vi "GetIdxString.vi"(10 "IdxArray":i32[](array[numeric]), 11 "StrArray":string[](array[string])) -> (7 "TrueArray":string[](array[string]))   [LabVIEW 2015]
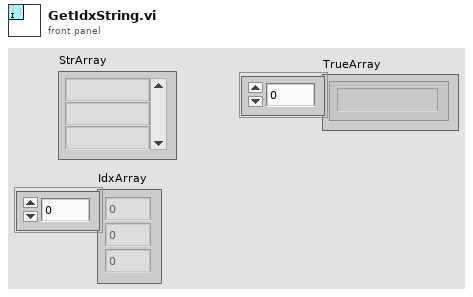
[diagram p1: front panel]
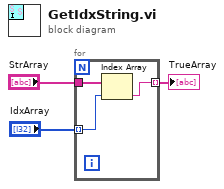
[diagram p0: block diagram]
diagram:
  n1 = for {
    tunnel: "StrArray" -> [w5]
    tunnel: "IdxArray" -> [w4] mode=indexing
    tunnel: [w6] -> w1 mode=indexing
    n2 = Index Array(array=w5, index=w4) -> (element=w6:string)
  }
  "TrueArray" <- w1
